vi "Get Symbol Information.vi"(8 "error in (no error)":errorcluster, 10 "Symbol Name":string, 11 "TwinCAT ADS in":refnum<class "TwinCAT ADS.lvclass">) -> (0 "error out":errorcluster, 1 ".NET Symbol Information":refnum<k24>, 3 "TwinCAT ADS out":refnum<class "TwinCAT ADS.lvclass">)   [LabVIEW 2018, in "TwinCAT ADS.lvclass"]
uses:
  TwinCAT ADS.lvclass
  TwinCAT.Ads
  TwinCAT ADS.lvclass/TwinCAT ADS.ctl
  Get Symbol Map.vi
  Format String.vi
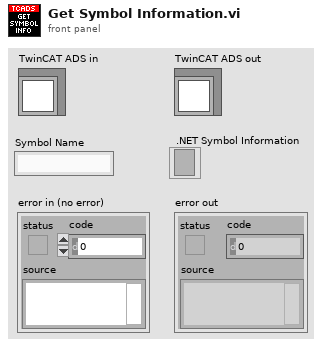
[diagram p1: front panel]
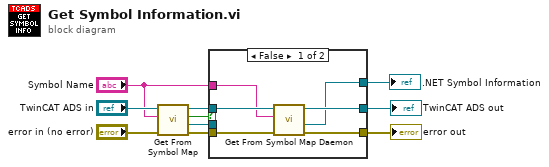
[diagram p0: block diagram]
diagram:
  n1 = call "Get From Symbol Map.vi"("error in (no error)"="error in (no error)", "Symbol Name"="Symbol Name", "TwinCAT ADS in"="TwinCAT ADS in") -> ("error out"=w2:errorcluster, ".NET Symbol Information"=w8:refnum<k24>, "Found?"=w7:bool, "TwinCAT ADS out"=w6:refnum<class "TwinCAT ADS.lvclass">)  [unwired: 5 in]
  n2 = case shown="False" w7 {
    tunnel: w8 -> [_ w17]
    tunnel: w6 -> [w16 w18]
    tunnel: w2 -> [w15 w19]
    tunnel: [w13 w19] -> w1
    tunnel: [w12 w18] -> w5
    tunnel: [w11 w17] -> w4
    tunnel: "Symbol Name" -> [w14 _]
    frame False {
      n3 = call "Get From Symbol Map Daemon.vi"("error in (no error)"=w15, "Symbol Name"=w14, "TwinCAT ADS in"=w16) -> ("error out"=w13:errorcluster, ".NET Symbol Information"=w11:refnum<k24>, "TwinCAT ADS out"=w12:refnum<class "TwinCAT ADS.lvclass">)  [unwired: 5 in, 1 out]
    }
    frame True {
    }
  }
  "error out" <- w1
  "TwinCAT ADS out" <- w5
  ".NET Symbol Information" <- w4
